vi "_002.vi"() -> ()   [LabVIEW 2024]
panel:
  out "K":dbl(slide) scale=-50.0..50.0
  out "C":dbl(slide) scale=0.0..500.0
  out "K":dbl(slide) scale=0.0..500.0
  out "F":dbl(slide) scale=0.0..100.0
  in  "F":dbl
  out "K":dbl
  in  "K":dbl
  out "C":dbl
  out "K":dbl
  in  "C":dbl
  out "F":dbl
  in  "C":dbl
  # "CONVERSION :"
  # "Celsious to Farenhiet :"
  # "Celsious to Kelvin :"
  # "Kelvin to Celsius :"
  # "Farenhiet to Kelvin :"
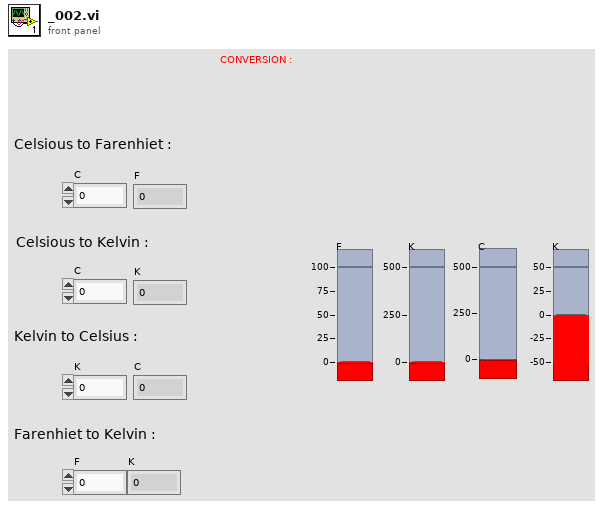
[diagram p1: front panel]
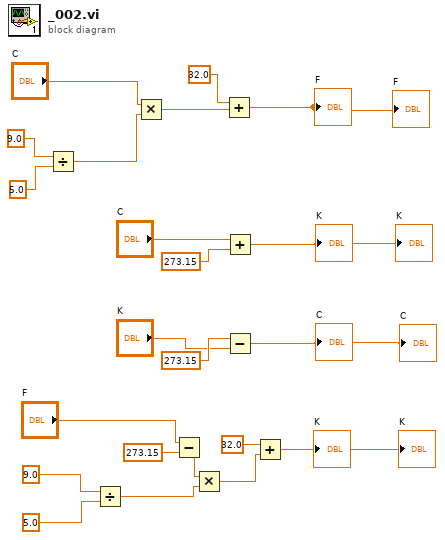
[diagram p0: block diagram]
diagram:
  n1 = Divide(x=9.0, y=5.0) -> (x/y=w19:dbl)
  n2 = Divide(x=9.0, y=5.0) -> (x/y=w7:dbl)
  n3 = Multiply(x="C", y=w19) -> (x*y=w18:dbl)
  n4 = Subtract(x="F", y=273.15) -> (x-y=w12:dbl)
  n5 = Multiply(x=w12, y=w7) -> (x*y=w6:dbl)
  n6 = Add(x=32.0, y=w18) -> (x+y=→"F" →"F":dbl)
  n7 = Add(x="C", y=273.15) -> (x+y=→"K" →"K":dbl)
  n8 = Subtract(x=273.15 ("y"), y="K") -> (x-y=→"C" →"C":dbl)
  n9 = Add(x=32.0, y=w6) -> (x+y=→"K" →"K":dbl)
